vi "write_summary_out.vi"(8 "# REACTORS":u32, 9 "REACTOR INDEX":u32, 10 "REACTOR ARRAY":T1, 11 "DATA FILE":path) -> ()   [LabVIEW 2013]
uses:
  main_machine/type_defs/reactors.ctl
  main_machine/type_defs/reactor.ctl
  <vilib>/Utility/file.llb/Write To Spreadsheet File (DBL).vi
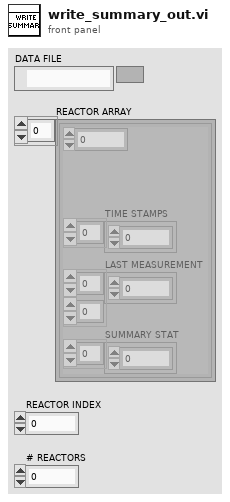
[diagram p1: front panel]
types:
  T1 = typedef "reactors.ctl" = cluster{i32, "TIME STAMPS":dbl[], "LAST MEASUREMENT":T2[][], "SUMMARY STAT":dbl[]}[]
  T2 = typedef "reactor.ctl" = dbl
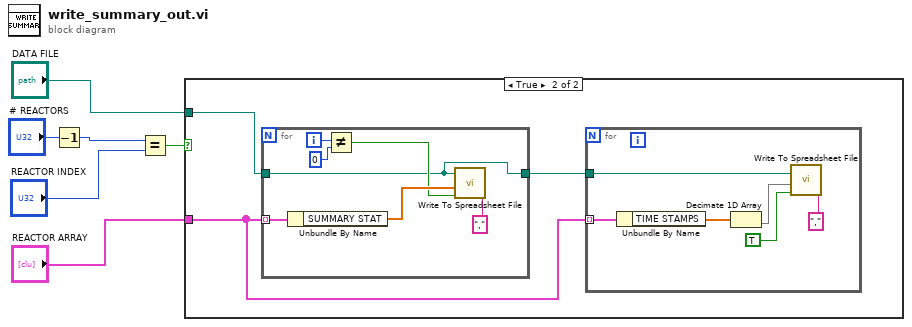
[diagram p0: block diagram]
diagram:
  n1 = Decrement(x="# REACTORS") -> (x-1=w1:u32)
  n2 = Equal?(x=w1, y="REACTOR INDEX") -> (x = y?=w2:bool)
  n3 = case shown="True" w2 {
    tunnel: "REACTOR ARRAY" -> [_ w7]
    tunnel: "DATA FILE" -> [_ w9]
    frame False {
    }
    frame True {
      n4 = for {
        tunnel: w7 -> [w22] mode=indexing
        tunnel: w9 -> [w16]
        tunnel: [w16] -> w8
        i -> [w17]
        n5 = Unbundle By Name(w22) -> ("SUMMARY STAT"=w21:dbl[])
        n6 = Not Equal?(x=w17, y=0) -> (x != y?=w18:bool)
        n7 = call-poly <vilib>:"Write To Spreadsheet File.vi"("delimiter (\\t)"="," ("delimiter (\\t)"), "append to file? (new file:F)"=w18, "1D data"=w21, "file path (dialog if empty)"=w16) -> ()  [unwired: 4 in, 1 out]
      }
      n8 = for {
        tunnel: w7 -> [w15] mode=indexing
        tunnel: w8 -> [w14]
        n9 = Unbundle By Name(w15) -> ("TIME STAMPS"=w12:dbl[])
        n10 = Decimate 1D Array(w12) -> (w11:dbl[])  [unwired: 1 out]
        n11 = call-poly <vilib>:"Write To Spreadsheet File.vi"("delimiter (\\t)"="," ("delimiter (\\t)"), "append to file? (new file:F)"=TRUE, "1D data"=w11, "file path (dialog if empty)"=w14) -> ()  [unwired: 4 in, 1 out]
      }
    }
  }
